vi "Auto HP indexer.vi"(11 "MechanismMetrics in":T1) -> (3 "MechanismMetrics in 2":T1)   [LabVIEW 2014]
uses:
  MechanismMetrics.ctl
  Lifter States.ctl
  Auto Lifter States.ctl
  <vilib>/Rock Robotics/WPI/Solenoid/WPI_SolenoidValue.ctl
  Lifter Hights.vi
  <vilib>/Rock Robotics/WPI/Solenoid/WPI_SolenoidSetEnum.vi
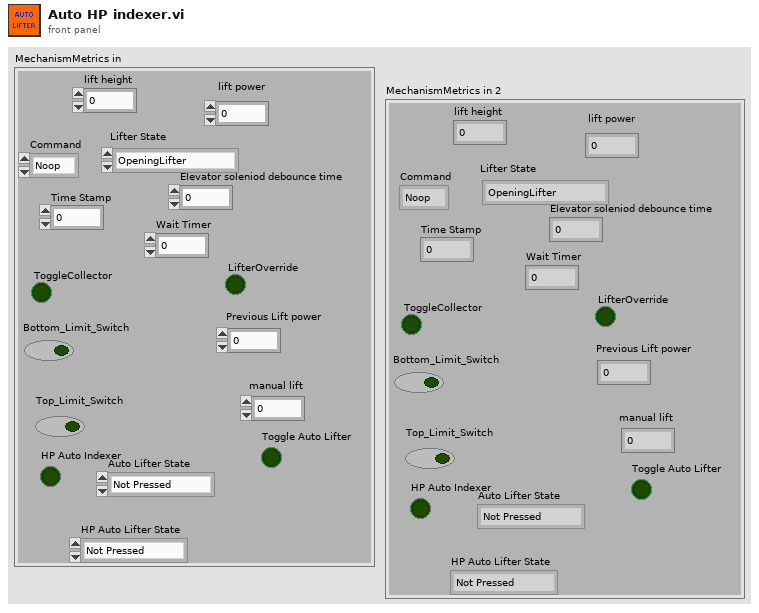
[diagram p1: front panel]
types:
  T1 = typedef "MechanismMetrics.ctl" = cluster{"lift height":dbl, "Command":enum16{"Noop", "Flagged"}, "Time Stamp":u32, "ToggleCollector":bool, "Bottom_Limit_Switch ":bool, "Top_Limit_Switch":bool, "lift power":dbl, "Elevator soleniod debounce time   ":dbl, "LifterOverride":bool, "Previous Lift power":dbl, "manual lift":dbl, "Lifter State":T2, "Auto Lifter State":T3, "Toggle Auto Lifter":bool, "Wait Timer":dbl, "HP Auto Indexer":bool, "HP Auto Lifter State":T3}
  T2 = typedef "Lifter States.ctl" = enum16{"OpeningLifter", "LifterOpen", "ClosingLifter", "LifterClosed"}
  T3 = typedef "Auto Lifter States.ctl" = enum16{"Not Pressed", "THE_END", "WAIT_FOR_RELEASE", "Press Detected", "To Release Stacked1", "To Collect", "Open Lifter", "WAIT", "Close", "To Stack1"}
  T4 = typedef "WPI_SolenoidValue.ctl" = enum16{"Off", "On", "Forward", "Reverse"}
  T5 = typedef "WPI_SolenoidDevRef.ctl" = cluster{"DevStatus":errorcluster, "Pneumatics Control Module":u8, "Forward Solenoid Channel":T6, "Reverse Solenoid Channel":T6}
  T6 = typedef "WPI_SolenoidChannel.ctl" = enum8{"Solenoid 0", "Solenoid 1", "Solenoid 2", "Solenoid 3", "Solenoid 4", "Solenoid 5", "Solenoid 6", "Solenoid 7", "Invalid"}
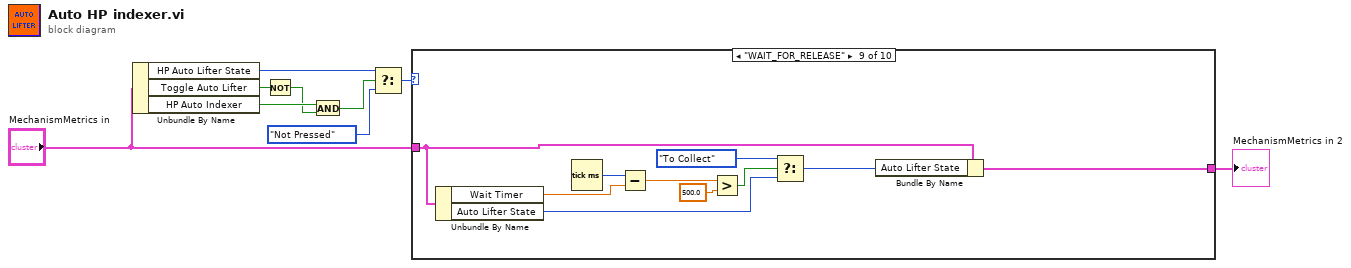
[diagram p0: block diagram]
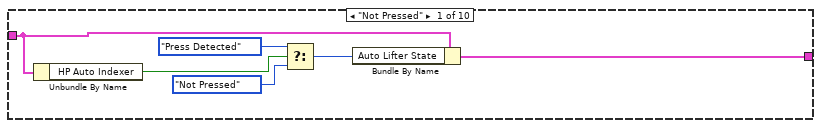
[diagram p2: hidden frame]
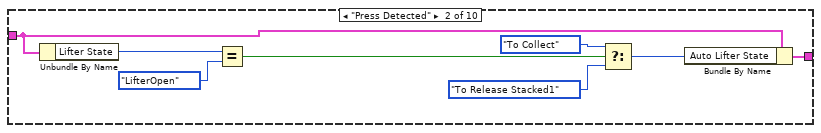
[diagram p3: hidden frame]
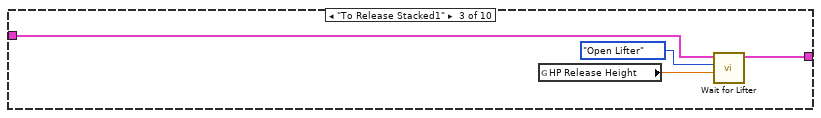
[diagram p4: hidden frame]
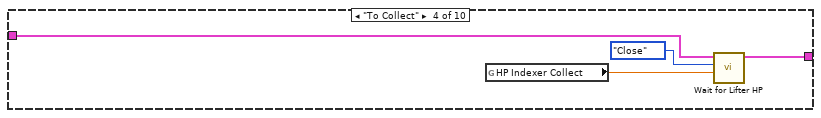
[diagram p5: hidden frame]
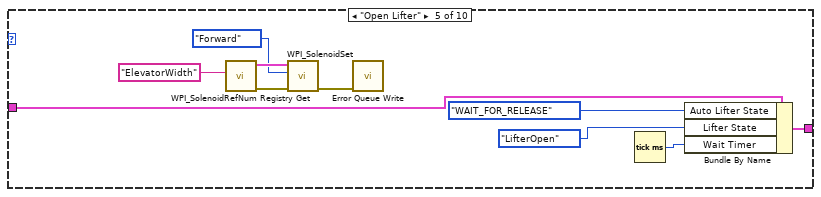
[diagram p6: hidden frame]
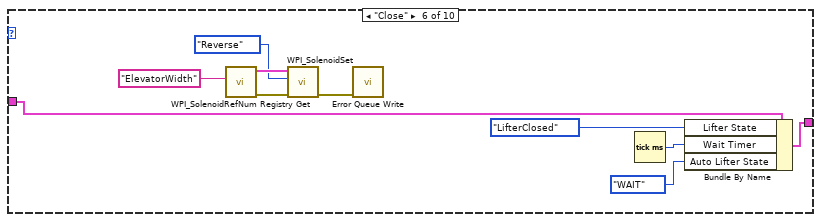
[diagram p7: hidden frame]
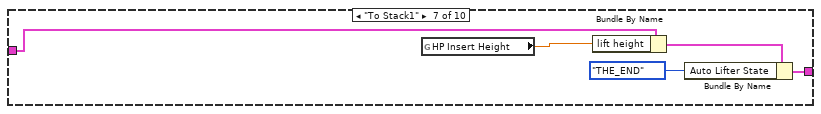
[diagram p8: hidden frame]
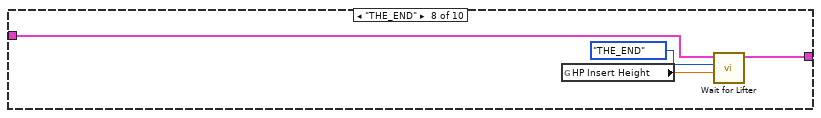
[diagram p9: hidden frame]
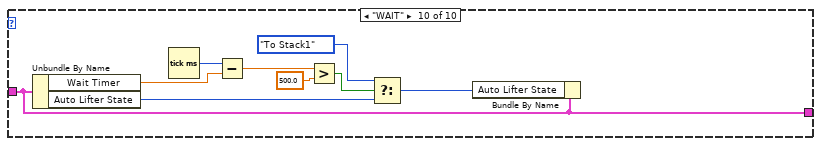
[diagram p10: hidden frame]
diagram:
  n1 = Unbundle By Name("MechanismMetrics in") -> ("HP Auto Lifter State"=w7:T3, "Toggle Auto Lifter"=w4:bool, "HP Auto Indexer"=w6:bool)
  n2 = Not(x=w4) -> (.not. x?=w3:bool)
  n3 = And(x=w6, y=w3) -> (x .and. y?=w5:bool)
  n4 = Select(t=w7, s=w5, f=Auto_Lifter_States."Not Pressed") -> (s? t:f=w1:T3)
  n5 = case shown="\"WAIT_FOR_RELEASE\"" w1 {
    tunnel: "MechanismMetrics in" -> [w12 w18 w25 w31 w34 w45 w56 w58 w70 w74]
    tunnel: [w10 w16 w24 w28 w33 w46 w54 w57 w69 w74] -> w9
    frame "Not Pressed" {
      n6 = Unbundle By Name(w12) -> ("HP Auto Indexer"=w13:bool)
      n7 = Select(t=Auto_Lifter_States."Press Detected", s=w13, f=Auto_Lifter_States."Not Pressed") -> (s? t:f=w11:T3)
      n8 = Bundle By Name(cluster=w12, "Auto Lifter State"=w11) -> (w10:T1)
    }
    frame "Press Detected" {
      n9 = Unbundle By Name(w18) -> ("Lifter State"=w23:T2)
      n10 = Equal?(x=w23, y=Lifter_States."LifterOpen" ("Lifter States")) -> (x = y?=w21:bool)
      n11 = Select(t=Auto_Lifter_States."To Collect", s=w21, f=Auto_Lifter_States."To Release Stacked1") -> (s? t:f=w17:T3)
      n12 = Bundle By Name(cluster=w18, "Auto Lifter State"=w17) -> (w16:T1)
    }
    frame "To Release Stacked1" {
      n13 = global read "Lifter Hights.vi" "HP Release Height"() -> (w27:dbl)
      n14 = call "Wait for Lifter.vi"("1 tote high"=w27, "Auto Lifter States"=Auto_Lifter_States."Open Lifter", "MechanismMetrics in in"=w25) -> ("MechanismMetrics out"=w24:T1)  [unwired: 8 in]
    }
    frame "To Collect" {
      n15 = global read "Lifter Hights.vi" "HP Indexer Collect"() -> (w29:dbl)
      n16 = call "Wait for Lifter HP.vi"("1 tote high"=w29, "Auto Lifter States"=Auto_Lifter_States."Close", "MechanismMetrics in in"=w31) -> ("MechanismMetrics out"=w28:T1)  [unwired: 8 in]
    }
    frame "Open Lifter" {
      n17 = call <vilib>:"WPI_SolenoidRefNum Registry Get.vi"("refnum name"="ElevatorWidth") -> ("error out"=w41:errorcluster, "SolenoidDevRef"=w40:T5)  [unwired: 9 in]
      n18 = call-poly <vilib>:"WPI_SolenoidSet.vi"("error in (no error)"=w41, "Value"=WPI_SolenoidValue."Forward", "SolenoidDevRef"=w40) -> ("error out"=w38:errorcluster)  [unwired: 7 in, 1 out]
      n19 = call "Error Queue Write.vi"("error in (no error)"=w38) -> ()  [unwired: 11 in]
      n20 = Tick Count (ms)() -> (millisecond timer value=w36:u32)
      n21 = Bundle By Name(cluster=w34, "Auto Lifter State"=Auto_Lifter_States."WAIT_FOR_RELEASE" ("f"), "Lifter State"=Lifter_States."LifterOpen" ("Lifter States"), "Wait Timer"=w36) -> (w33:T1)
    }
    frame "Close" {
      n22 = call <vilib>:"WPI_SolenoidRefNum Registry Get.vi"("refnum name"="ElevatorWidth") -> ("error out"=w49:errorcluster, "SolenoidDevRef"=w50:T5)  [unwired: 9 in]
      n23 = call-poly <vilib>:"WPI_SolenoidSet.vi"("error in (no error)"=w49, "Value"=WPI_SolenoidValue."Reverse", "SolenoidDevRef"=w50) -> ("error out"=w51:errorcluster)  [unwired: 7 in, 1 out]
      n24 = call "Error Queue Write.vi"("error in (no error)"=w51) -> ()  [unwired: 11 in]
      n25 = Tick Count (ms)() -> (millisecond timer value=w43:u32)
      n26 = Bundle By Name(cluster=w45, "Lifter State"=Lifter_States."LifterClosed" ("Lifter States"), "Wait Timer"=w43, "Auto Lifter State"=Auto_Lifter_States."WAIT" ("f")) -> (w46:T1)
    }
    frame "To Stack1" {
      n27 = global read "Lifter Hights.vi" "HP Insert Height"() -> (w52:dbl)
      n28 = Bundle By Name(cluster=w56, "lift height"=w52) -> (w55:T1)
      n29 = Bundle By Name(cluster=w55, "Auto Lifter State"=Auto_Lifter_States."THE_END" ("Auto Lifter States")) -> (w54:T1)
    }
    frame "THE_END" {
      n30 = global read "Lifter Hights.vi" "HP Insert Height"() -> (w59:dbl)
      n31 = call "Wait for Lifter.vi"("1 tote high"=w59, "Auto Lifter States"=Auto_Lifter_States."THE_END", "MechanismMetrics in in"=w58) -> ("MechanismMetrics out"=w57:T1)  [unwired: 8 in]
    }
    frame "WAIT_FOR_RELEASE" {
      n32 = Unbundle By Name(w70) -> ("Wait Timer"=w62:dbl, "Auto Lifter State"=w65:T3)
      n33 = Tick Count (ms)() -> (millisecond timer value=w63:u32)
      n34 = Subtract(x=w63, y=w62) -> (x-y=w61:dbl)
      n35 = Greater?(x=w61, y=500.0) -> (0:w67:bool)
      n36 = Select(t=Auto_Lifter_States."To Collect", s=w67, f=w65) -> (s? t:f=w66:T3)
      n37 = Bundle By Name(cluster=w70, "Auto Lifter State"=w66) -> (w69:T1)
    }
    frame "WAIT" {
      n38 = Unbundle By Name(w74) -> ("Wait Timer"=w72:dbl, "Auto Lifter State"=w76:T3)
      n39 = Tick Count (ms)() -> (millisecond timer value=w73:u32)
      n40 = Subtract(x=w73, y=w72) -> (x-y=w71:dbl)
      n41 = Greater?(x=w71, y=500.0) -> (0:w78:bool)
      n42 = Select(t=Auto_Lifter_States."To Stack1", s=w78, f=w76) -> (s? t:f=w77:T3)
      n43 = Bundle By Name(cluster=w74, "Auto Lifter State"=w77) -> ()  [unwired: 1 out]
    }
  }
  "MechanismMetrics in 2" <- w9
